vi "温度上下限布尔报警文本提示.vi"() -> ()   [LabVIEW 2018]
panel:
  out "历史温度波形图表":dbl(graph)
  out "文本提示":string
  out "当前温度":dbl
  out "温度计":dbl(slide) scale=0.0..100.0
  out "低温提示":bool
  out "高温提示":bool
  in  "温度报警下限":dbl=10.0
  in  "温度报警上限":dbl=40.0
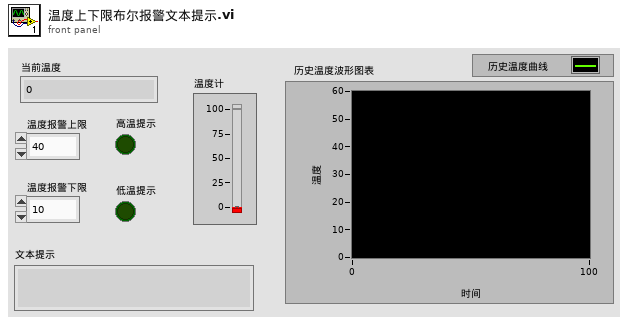
[diagram p1: front panel]
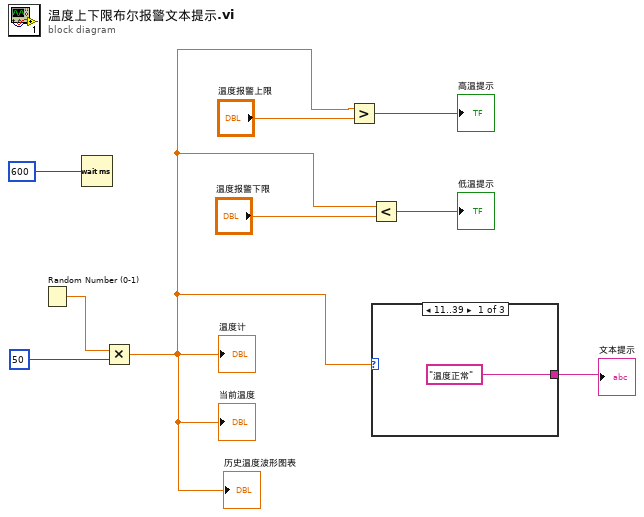
[diagram p0: block diagram]
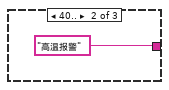
[diagram p2: hidden frame]
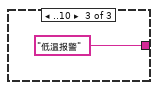
[diagram p3: hidden frame]
diagram:
  n1 = Random Number (0-1)() -> (number: 0 to 1=w5:dbl)
  n2 = Wait (ms)(milliseconds to wait=600) -> ()  [unwired: 1 out]
  n3 = Multiply(x=w5, y=50) -> (x*y=w1:dbl)
  "温度计" <- w1
  "当前温度" <- w1
  "历史温度波形图表" <- w1
  n4 = Greater?(x=w1, y="温度报警上限") -> (0:→"高温提示":bool)
  n5 = Less?(x=w1, y="温度报警下限") -> (x < y?=→"低温提示":bool)
  n6 = case shown="11..39" w1 {
    tunnel: ["温度正常" "高温报警" "低温报警"] -> w2
    frame 11..39 {
    }
    frame 40.. {
    }
    frame ..10 {
    }
  }
  "文本提示" <- w2
